vi "Compare Scalar Clusters.vi"(1 "Target bitfile scalars in":T1[](array[typedef]), 2 "Reference bitfile scalars in":T1[](array[typedef])) -> (0 "Equal ?":bool)   [LabVIEW 2018, in "FPGA Addon Scripting API Unit Tests.lvclass"]
uses:
  FPGA Addon Scripting API Unit Tests.lvclass
  APIs/Scripting API/TypeDefs/Output Scalar Data.ctl
  Addon/Addon Shared/Types/Data Type.ctl
  Addon/Addon Shared/FPGA Addon Shared.lvlib
  APIs/Scripting API/Scripting API.lvlib
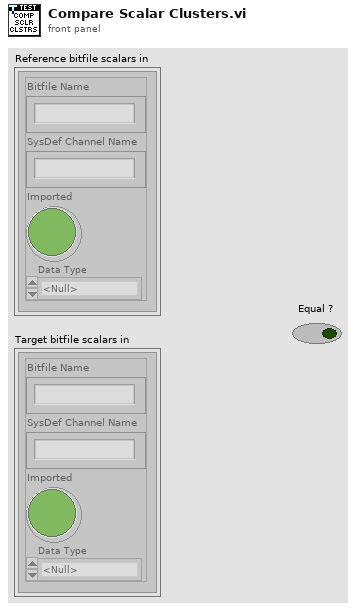
[diagram p1: front panel]
types:
  T1 = typedef "Scripting API.lvlib/Output Scalar Data.ctl" = cluster{"Bitfile Name":string, "SysDef Channel Name":string, "Imported":bool, "Data Type":T2}
  T2 = typedef "FPGA Addon Shared.lvlib/Data Type.ctl" = enum8{"<Null>", "I8", "I16", "I32", "I64", "U8", "U16", "U32", "U64", "SGL", "Boolean", "Analog PWM In Settings", "Analog PWM In", "Digital PWM In Settings", "Digital PWM In", "Digital PWM Out", "Sine Out", "FXP+/-24.5", "FXP+/-16.5", "FXP+/-32.8", "FXP+/-64.32", "FXP+/-16.7", "FXP+/-20.5", "FXP+/-27.5", "FXP+/-32.16", "FXP+16.3", "FXP+18.3", "Digital Static In", "Digital Static Out", "Digital Static In Settings", "Digital WSS Out", "Quad Encoder Settings", "Quad Encoder In", "Group"}
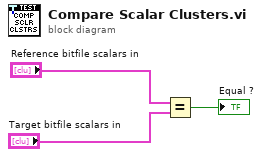
[diagram p0: block diagram]
diagram:
  n1 = Equal?(x="Reference bitfile scalars in", y="Target bitfile scalars in") -> (x = y?=→"Equal ?":bool)
